vi "抓圓.vi"(0 "Image In":T6, 1 "Process":T9(ring), 2 "Optimized Mode":bool, 5 "ROI":T5, 7 "Coordinate System":T4 {"Measurement System"."Axis Reference" items=["Direct", "Indirect"]; "Measurement System"."Angle (deg)" format="%.2f"; "Measurement System"."Origin"."Y" format="%.2f"; "Measurement System"."Origin"."X" format="%.2f"; "Reference System"."Axis Reference" items=["Direct", "Indirect"]; "Reference System"."Angle (deg)" format="%.2f"; "Reference System"."Origin"."Y" format="%.2f"; "Reference System"."Origin"."X" format="%.2f"}, 9 "Gap":i32=10 min=1 max=300, 11 "error In":errorcluster, 12 "Options":T3={"Search Direction"=0, "Edge Options"={"Edge Polarity"=0, "Kernel Size"=3, "Width"=3, "Minimum Edge Strength"=10.0, "Interpolation Type"=enum."Bilinear Fixed", "Data Processing Method"=enum."Average"}, "Show Search Area"=FALSE, "Show Search Lines"=FALSE, "Show Edges Found"=FALSE, "Show Result"=TRUE, "Search Area Color"=65280, "Search Lines Color"=255, "Edge Locations Color"=16776960, "Result Color"=16711680, "Overlay Group Name"=""} {"Edge Options"."Edge Polarity" items=["All Edges", "Rising Edges", "Falling Edges"]; "Edge Options"."Minimum Edge Strength" format="%.2f"; "Edge Options"."Width" step=2; "Edge Options"."Kernel Size" step=2; "Search Direction" items=["Outer to Inner", "Inner to Outer"]}, 13 "Point Diameter (5)":u32=5 min=3 max=1000) -> (4 "Imag e Out":T6, 6 "Line Profile":T7(graph), 8 "Gradient Information":dbl[][](graph), 14 "Ellipse":T8 {"Minor Axis"."Point 2"."Y" format="%.2f"; "Minor Axis"."Point 2"."X" format="%.2f"; "Minor Axis"."Point 1"."Y" format="%.2f"; "Minor Axis"."Point 1"."X" format="%.2f"; "Major Axis"."Point 2"."Y" format="%.2f"; "Major Axis"."Point 2"."X" format="%.2f"; "Major Axis"."Point 1"."Y" format="%.2f"; "Major Axis"."Point 1"."X" format="%.2f"; "Center"."Y" format="%.2f"; "Center"."X" format="%.2f"}, 15 "error out":errorcluster)   [LabVIEW 2015]
uses:
  <vilib>/vision/Image Controls.llb/IMAQ Image.ctl
  <vilib>/vision/Measure.llb/Edge Options.ctl
  <vilib>/vision/Measure.llb/Edge Polarity.ctl
  <vilib>/Analysis/coordinate.llb/2D Cartesian Coordinate Rotation (Scalar).vi
  <vilib>/vision/NI_Vision_Development_Module.lvlib
  <vilib>/Analysis/NI_AALPro.lvlib
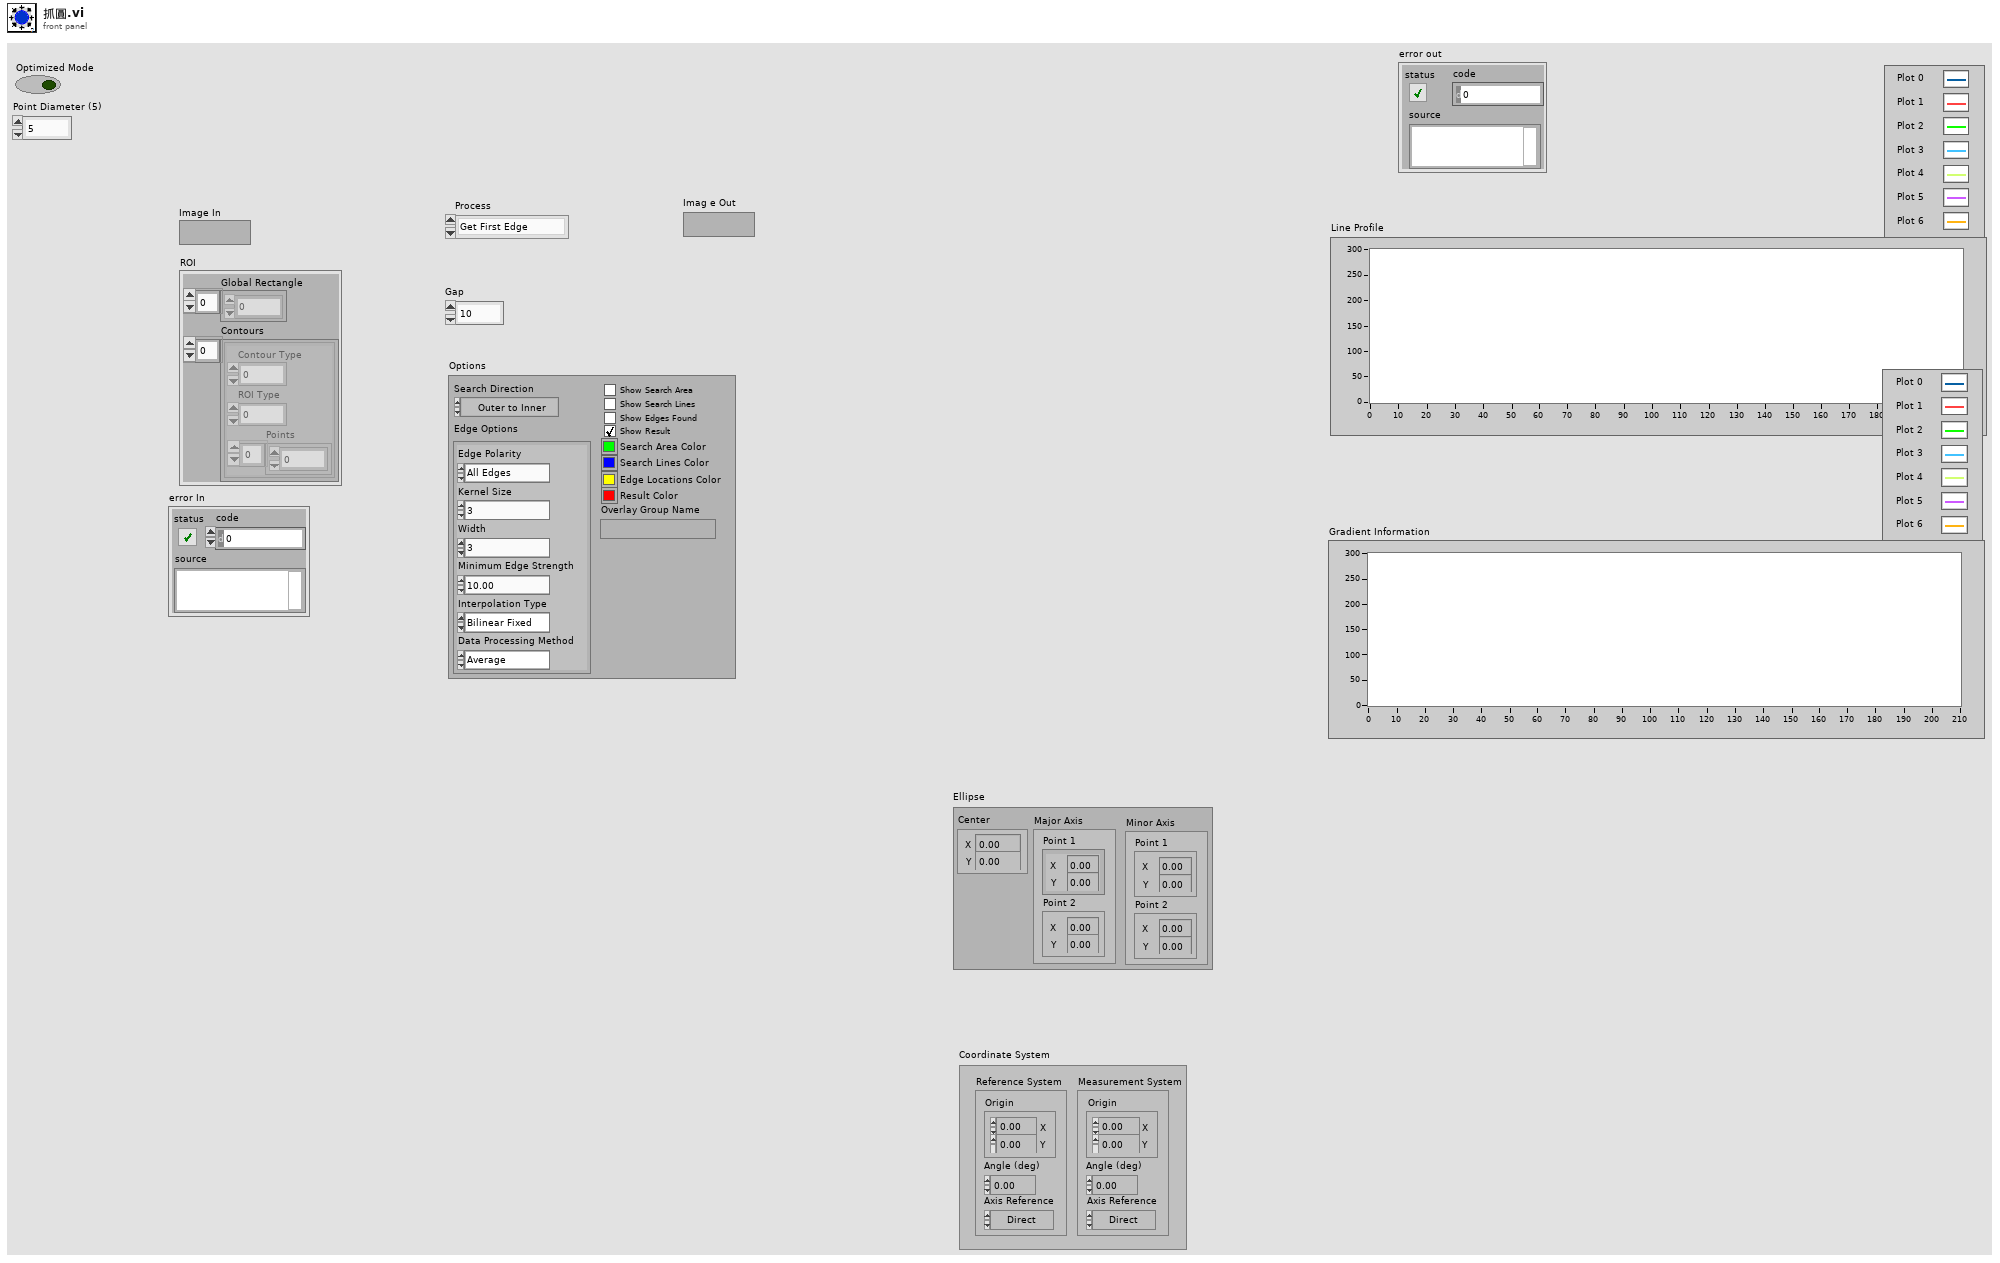
[diagram p1: front panel]
types:
  T1 = typedef "Edge Options.ctl" = cluster{"Edge Polarity":T2, "Kernel Size":u32, "Width":u32, "Minimum Edge Strength":sgl, "Interpolation Type":enum32{"Zero Order", "Bilinear", "Quadratic", "Cubic", "Bilinear Fixed"}, "Data Processing Method":enum32{"Average", "Median"}}
  T2 = typedef "Edge Polarity.ctl" = u32
  T3 = cluster{"Search Direction":u32, "Edge Options":T1, "Show Search Area":bool, "Show Search Lines":bool, "Show Edges Found":bool, "Show Result":bool, "Search Area Color":u32, "Search Lines Color":u32, "Edge Locations Color":u32, "Result Color":u32, "Overlay Group Name":string}
  T4 = typedef "IMAQ Coordinate System" = cluster{"Reference System":cluster{"Origin":cluster{"X":sgl, "Y":sgl}, "Angle (deg)":sgl, "Axis Reference":u32}, "Measurement System":cluster{"Origin":cluster{"X":sgl, "Y":sgl}, "Angle (deg)":sgl, "Axis Reference":u32}}
  T5 = cluster{"Global Rectangle":i32[], "Contours":cluster{"Contour Type":u32, "ROI Type":u32, "Points":i32[]}[]}
  T6 = typedef "IMAQ Image.ctl" = refnum<image>
  T7 = cluster{"x0":sgl, "dx":sgl, "Pixels Line":sgl[]}[]
  T8 = cluster{"Center":cluster{"X":sgl, "Y":sgl}, "Major Axis":cluster{"Point 1":cluster{"X":sgl, "Y":sgl}, "Point 2":cluster{"X":sgl, "Y":sgl}}, "Minor Axis":cluster{"Point 1":cluster{"X":sgl, "Y":sgl}, "Point 2":cluster{"X":sgl, "Y":sgl}}}
  T9 = enum16{"Get First Edge", "Get First + Last Edge", "Get All Edges", "Get Best Edge"}
  T10 = typedef "IMAQ Point" = cluster{"X":sgl, "Y":sgl}
  T11 = typedef "IMAQ Line" = cluster{"Start X":i32, "Start Y":i32, "End X":i32, "End Y":i32}
  T12 = cluster{"Point 1":cluster{"x":dbl, "y":dbl}, "Point 2":cluster{"x":dbl, "y":dbl}}
  T13 = cluster{"Origin":cluster{"X":sgl, "Y":sgl}, "Angle (deg)":sgl, "Axis Reference":u32}
  T14 = typedef "ROI Descriptor" = cluster{"Global Rectangle":i32[], "Contours":cluster{"ID":enum32{"External", "Internal"}, "Type":u32, "Coordinates":i32[]}[]}
  T15 = typedef "IMAQ Circle" = cluster{"Center X":i32, "Center Y":i32, "Inner Radius":i32, "Outer Radius":i32, "Start Angle":dbl, "End Angle":dbl}
  T16 = typedef "Edge New.ctl" = cluster{"Location (Pixel)":cluster{"X":sgl, "Y":sgl}, "Location (Real-World)":cluster{"X":sgl, "Y":sgl}, "Distance (Pixel)":dbl, "Distance (Real-World)":dbl, "Strength":dbl, "Noise":dbl, "Rising?":bool}
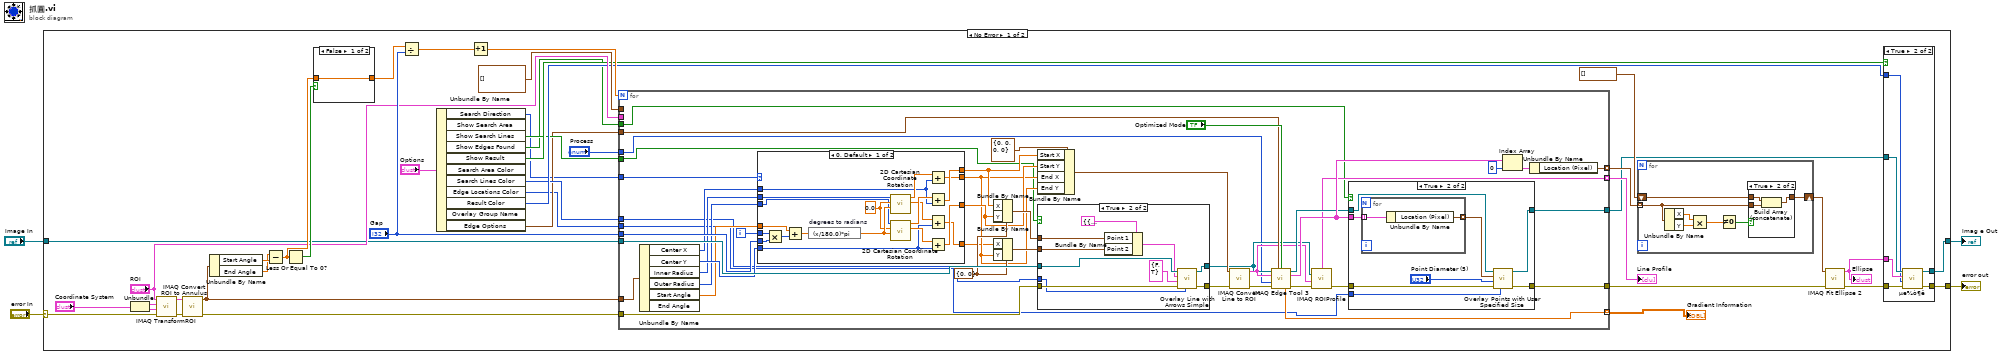
[diagram p0: block diagram]
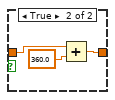
[diagram p3: hidden frame]
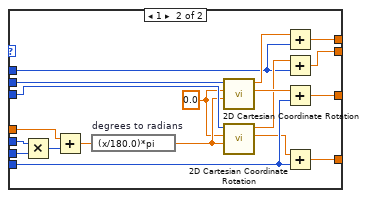
[diagram p7: hidden frame]
diagram:
  n1 = case shown="No Error" "error In" {
    selector: "error In" -> [w18 w173]
    tunnel: [w20 w173] -> w4
    tunnel: "Image In" -> [w16 w172]
    tunnel: [w15 w172] -> w1
    frame No Error {
      n2 = Unbundle("Coordinate System") -> ("Reference System"=w28:T13, "Measurement System"=w27:T13)
      n3 = call "IMAQ TransformROI"("error in (no error)"=w18, "New Reference"=w27, "Base Reference"=w28, "ROI Descriptor"="ROI") -> ("error out"=w24:errorcluster, "ROI Descriptor out"=w25:T14)  [unwired: 6 in]
      n4 = call "IMAQ Convert ROI to Annulus"("error in (no error)"=w24, "ROI Descriptor"=w25) -> ("error out"=w12:errorcluster, "Annulus"=w23:T15)  [unwired: 7 in]
      n5 = Unbundle By Name(w23) -> ("Start Angle"=w34:dbl, "End Angle"=w21:dbl)
      n6 = Subtract(x=w21, y=w34) -> (x-y=w30:dbl)
      n7 = Less Or Equal To 0?(x=w30) -> (x <= 0?=w31:bool)
      n8 = case shown="False" w31 {
        tunnel: w30 -> [w53 w55]
        tunnel: [w53 w54] -> w29
        frame False {
        }
        frame True {
          n9 = Add(x=w55, y=360.0) -> (x+y=w54:dbl)
        }
      }
      n10 = Divide(x=w29, y="Gap") -> (x/y=w35:dbl)
      n11 = Unbundle By Name("Options") -> ("Search Direction"=w6:u32, "Show Search Lines"=w11:bool, "Show Edges Found"=w7:bool, "Show Result"=w14:bool, "Search Lines Color"=w10:u32, "Edge Locations Color"=w8:u32, "Result Color"=w13:u32, "Edge Options"=w9:T1)  [unwired: 3 out]
      n12 = Increment(x=w35) -> (x+1=w41:dbl)
      n13 = for {
        N: w41 -> [_]
        tunnel: w6 -> [w95]
        tunnel: [w105] -> w32
        tunnel: w16 -> [w96]
        tunnel: "ROI" -> [_]
        tunnel: [w104] -> w37
        tunnel: "Process" -> [w68]
        tunnel: w9 -> [w103]
        tunnel: [w102] -> w40 mode=indexing
        tunnel: [w101] -> w5 mode=indexing
        tunnel: [w100] -> w39 mode=indexing
        tunnel: "Gap" -> [w94]
        tunnel: w23 -> [w92]
        tunnel: T10[] [] ("Rectangle Points") -> [_]
        tunnel: w12 -> [w73]
        tunnel: w11 -> [w72]
        tunnel: w10 -> [w71]
        tunnel: w8 -> [w70]
        tunnel: w7 -> [w69]
        i -> [w93]
        w89 = cluster{"X":i32, "Y":i32} {"X"=0, "Y"=0} ("Start Point")
        n14 = Unbundle By Name(w92) -> ("Center X"=w78:i32, "Center Y"=w77:i32, "Inner Radius"=w76:i32, "Outer Radius"=w75:i32, "Start Angle"=w74:dbl)  [unwired: 1 out]
        n15 = case shown="0, Default" w95 {
          tunnel: w77 -> [w136 w171]
          tunnel: w76 -> [w135 w170]
          tunnel: w75 -> [w134 w169]
          tunnel: w74 -> [w139 w168]
          tunnel: w94 -> [w137 w167]
          tunnel: w93 -> [w138 w158]
          tunnel: [w144 w153] -> w84
          tunnel: [w142 w157] -> w82
          tunnel: w78 -> [w140 w156]
          tunnel: [w141 w155] -> w81
          tunnel: [w143 w154] -> w83
          frame 0, Default {
            w147 = 0.0 ("y")
            n16 = Multiply(x=w138, y=w137) -> (x*y=w146:i32)
            n17 = Add(x=w139, y=w146) -> (x+y=w145:dbl)
            n18 = expression code="(x/180.0)*pi" "degrees to radians"(w145) -> (w148:dbl)
            n19 = call-poly <vilib>:"2D Cartesian Coordinate Rotation.vi"("theta"=w148, "y"=w147, "x"=w135) -> ("y out"=w150:dbl, "x out"=w149:dbl)  [unwired: 6 in, 1 out]
            n20 = call-poly <vilib>:"2D Cartesian Coordinate Rotation.vi"("theta"=w148, "y"=w147, "x"=w134) -> ("y out"=w151:dbl, "x out"=w152:dbl)  [unwired: 6 in, 1 out]
            n21 = Add(x=w149, y=w140) -> (x+y=w141:dbl)
            n22 = Add(x=w152, y=w140) -> (x+y=w144:dbl)
            n23 = Add(x=w150, y=w136) -> (x+y=w142:dbl)
            n24 = Add(x=w151, y=w136) -> (x+y=w143:dbl)
          }
          frame 1 {
            w161 = 0.0 ("y")
            n25 = Multiply(x=w158, y=w167) -> (x*y=w160:i32)
            n26 = Add(x=w168, y=w160) -> (x+y=w159:dbl)
            n27 = expression code="(x/180.0)*pi" "degrees to radians"(w159) -> (w162:dbl)
            n28 = call-poly <vilib>:"2D Cartesian Coordinate Rotation.vi"("theta"=w162, "y"=w161, "x"=w170) -> ("y out"=w165:dbl, "x out"=w166:dbl)  [unwired: 6 in, 1 out]
            n29 = call-poly <vilib>:"2D Cartesian Coordinate Rotation.vi"("theta"=w162, "y"=w161, "x"=w169) -> ("y out"=w164:dbl, "x out"=w163:dbl)  [unwired: 6 in, 1 out]
            n30 = Add(x=w166, y=w156) -> (x+y=w153:dbl)
            n31 = Add(x=w163, y=w156) -> (x+y=w155:dbl)
            n32 = Add(x=w165, y=w171) -> (x+y=w154:dbl)
            n33 = Add(x=w164, y=w171) -> (x+y=w157:dbl)
          }
        }
        n34 = Bundle By Name(cluster=w89, "X"=w84, "Y"=w83) -> (w87:cluster{"X":i32, "Y":i32})
        n35 = Bundle By Name(cluster=w89, "X"=w81, "Y"=w82) -> (w88:cluster{"X":i32, "Y":i32})
        n36 = Bundle By Name(cluster=T11 {"Start X"=0, "Start Y"=0, "End X"=0, "End Y"=0} ("Line"), "Start X"=w84, "Start Y"=w83, "End X"=w81, "End Y"=w82) -> (w90:T11)
        n37 = case shown="True" w72 {
          tunnel: w96 -> [w123 w133]
          tunnel: w88 -> [_ w132]
          tunnel: w87 -> [_ w131]
          tunnel: [w123 w127] -> w86
          tunnel: [w122 w126] -> w85
          tunnel: w73 -> [w122 w125]
          tunnel: w71 -> [_ w124]
          frame False {
          }
          frame True {
            n38 = Bundle By Name(cluster=T12 {"Point 1"={"x"=50.0, "y"=50.0}, "Point 2"={"x"=70.0, "y"=70.0}} ("Line Coordinates"), "Point 1"=w131, "Point 2"=w132) -> (w128:T12)
            n39 = call "Overlay Line with Arrows Simple.vi"("Color"=w124, "error in"=w125, "Arrows"=cluster{"Start point":bool, "End point":bool} {"Start point"=FALSE, "End point"=TRUE}, "Line Coordinates"=w128, "Image In"=w133) -> ("error out"=w126:errorcluster, "Image Out"=w127:T6)  [unwired: 5 in]
          }
        }
        n40 = call "IMAQ Convert Line to ROI"("error in (no error)"=w85, "Line"=w90) -> ("error out"=w98:errorcluster, "ROI Descriptor"=w97:T14)  [unwired: 7 in]
        n41 = call "IMAQ Edge Tool 3"("Image"=w86, "Edge Options"=w103, "Optimized Mode"="Optimized Mode", "ROI Descriptor"=w97, "Process"=w68, "error in (no error)"=w98) -> ("Image (duplicate)"=w106:T6, "Edge Information"=w109:T16[], "Gradient Values"=w101:dbl[], "error out"=w99:errorcluster)  [unwired: 5 in, 1 out]
        n42 = call "IMAQ ROIProfile"("error in (no error)"=w99, "ROI Descriptor"=w97, "Image"=w86) -> ("error out"=w108:errorcluster, "ROI Graph"=w102:cluster{"x0":sgl, "dx":sgl, "Pixels Line":sgl[]})  [unwired: 1 in, 3 out]
        n43 = case shown="True" w69 {
          tunnel: w109 -> [_ w119]
          tunnel: w108 -> [w110 w118]
          tunnel: w106 -> [w111 w117]
          tunnel: [w111 w116] -> w105
          tunnel: [w110 w115] -> w104
          tunnel: w70 -> [_ w112]
          frame False {
          }
          frame True {
            n44 = for {
              tunnel: w119 -> [w121] mode=indexing
              tunnel: [w120] -> w114 mode=indexing
              n45 = Unbundle By Name(w121) -> ("Location (Pixel)"=w120:cluster{"X":sgl, "Y":sgl})
            }
            n46 = call "Overlay Points with User Specified Size.vi"("Color"=w112, "error in"=w118, "Point Diameter (5)"="Point Diameter (5)", "Points"=w114, "Image In"=w117) -> ("error out"=w115:errorcluster, "Image Out"=w116:T6)  [unwired: 5 in]
          }
        }
        n47 = Index Array(array=w109, index=0) -> (element=w79:T16)
        n48 = Unbundle By Name(w79) -> ("Location (Pixel)"=w100:cluster{"X":sgl, "Y":sgl})
      }
      "Line Profile" <- w40
      "Gradient Information" <- w5
      n49 = for {
        tunnel: w39 -> [w59] mode=indexing
        shift-right: [w58] -> w38
        shift-left: cluster{"X":sgl, "Y":sgl}[] [] -> [w57]
        n50 = Unbundle By Name(w59) -> ("X"=w63:sgl, "Y"=w62:sgl)
        n51 = Multiply(x=w63, y=w62) -> (x*y=w61:sgl)
        n52 = Not Equal To 0?(x=w61) -> (x != 0?=w60:bool)
        n53 = case shown="True" w60 {
          tunnel: w59 -> [_ w67]
          tunnel: [w64 w66] -> w58
          tunnel: w57 -> [w64 w65]
          frame False {
          }
          frame True {
            n54 = Build Array (concatenate)(w65, w67) -> (w66:cluster{"X":sgl, "Y":sgl}[])
          }
        }
      }
      n55 = call "IMAQ Fit Ellipse 2"("error in (no error)"=w37, "Radial Points"=w38) -> ("error out"=w19:errorcluster, "Ellipse"=w33:T8)  [unwired: 4 in, 4 out]
      "Ellipse" <- w33
      n56 = case shown="True" w14 {
        tunnel: w33 -> [_ w52]
        tunnel: w32 -> [w46 w51]
        tunnel: [w45 w50] -> w20
        tunnel: w19 -> [w45 w49]
        tunnel: [w46 w48] -> w15
        tunnel: w13 -> [_ w47]
        frame False {
        }
        frame True {
          n57 = call "µe¾ò¶ê.vi"("error in (no error)"=w49, "Color"=w47, "Ellipse"=w52, "Image In"=w51) -> ("error out"=w50:errorcluster, "Image"=w48:T6)  [unwired: 6 in]
        }
      }
    }
    frame Error {
    }
  }
  "error out" <- w4
  "Imag e Out" <- w1
